vi "Data FIFO Probe Boolean.vi"(8 "Valid":bool=TRUE, 11 "Input":bool) -> (3 "Array":bool[](array[boolean]))   [LabVIEW 2012]
doc: "This VI is used to probe Array of data on FPGA during simulation"
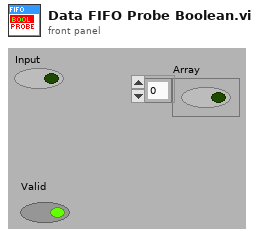
[diagram p1: front panel]
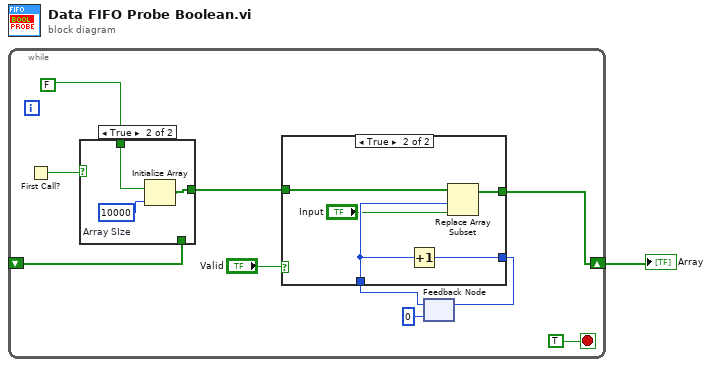
[diagram p0: block diagram]
diagram:
  n1 = while {
    shift-right: [w11] -> w1
    shift-left: _ -> [w9]
    stop <- TRUE stop-if-true
    n2 = First Call?() -> (First Call?: T/F=w7:bool)
    n3 = case shown="True" w7 {
      tunnel: [w19 w21] -> w10
      tunnel: w9 -> [w19 _]
      tunnel: FALSE -> [_ w20]
      frame False {
      }
      frame True {
        w22 = 10000  # Array SIze
        n4 = Initialize Array(w20, w22) -> (w21:bool[])
      }
    }
    n5 = feedback #1(u32 0) -> (w4:u32)
    n6 = case shown="True" "Valid" {
      tunnel: [w13 w18] -> w11
      tunnel: w10 -> [w13 w17]
      tunnel: w4 -> [w12 w15]
      tunnel: [w12 w16] -> w3
      frame False {
      }
      frame True {
        n7 = Increment(x=w15) -> (x+1=w16:u32)
        n8 = Replace Array Subset(array=w17, new element="Input", index=w15) -> (w18:bool[])
      }
    }
    n9 = feedback-in #1(w3) -> ()
  }
  "Array" <- w1
